vi "GUI_HTT_CTRLv4.vi"() -> ()   [LabVIEW 2020]
uses:
  Shared/GUI_Template/GUI_master/tcp_new_data_event.ctl
  Shared/GUI_Template/GUI_master/tcp new data cluster.ctl
  GUI_TestStand/Fire button.ctl
  <vilib>/Platform/browser.llb/Open URL in Default Browser (string).vi
panel:
  in  "LogEpilog":bool caption="LogTable"
  in  "New Google\nExpLog for new day?":bool=TRUE
  in  "LogTable":bool
  in  "PicoL2":bool caption="PicoL GUI"
  in  "1Wire B GUI":bool caption="PicoL GUI"
  out "fire::12":string="fire" caption="fire"
  in  "Wavelength.Channel0::14":enum16{"248", "355", "532", "800", "2940"}(ring)=enum."532"
  in  "Wavelength.Channel1::14":enum16{"248", "355", "532", "800", "2940"}(ring)=enum."800"
  in  "Wavelength.Channel0::13":enum16{"532", "800"}(ring)=enum."800"
  in  "EnergyRange.Channel0::14":T1(ring)=enum."400mJ"
  in  "EnergyRange.Channel1::14":T1(ring)=enum."400mJ"
  in  "EnergyRange.Channel0::13":T2(ring)=enum."200mJ"
  in  "energy.channel 1::14":dbl caption="Energy Gaia" min=0.0 max=200.0 format="%#_13g"
  out "Energy (J)":dbl
  in  "Multiplicator":dbl=15.3
  in  "GUIdevice 14":string="HTT-Energy-S-G"
  in  "Multiplicator":dbl=66.6
  in  "Multiplicator Scatter":dbl=100.0
  out "Energy Scatter (J)":dbl
  out "Energy (J)":dbl
  in  "energy.channel 0::13":dbl caption="Energy Drive" min=0.0 max=10.0 format="%#_13g"
  in  "energy.channel 0::14":dbl caption="Energy Scatter" min=0.0 max=20.0 format="%#_13g"
  in  "GUIdevice 13":string="HTT-Energy-D"
  in  "IR Pt Exp And Comp":bool caption="PicoL GUI"
  in  "Position.Axis 2::10":dbl caption="y/vert." min=-6000.0 max=6000.0
  in  "Position.Axis 3::10":dbl caption="Scatter Mode z" min=-20.0 max=20.0
  in  "Position.Axis 1::10":dbl caption="x/hor." min=-150.0 max=150.0
  in  "Position.Axis 2::11":dbl caption="Translation" min=-50.0 max=50.0
  in  "Position.Axis 3::11":dbl caption="Rotation G1" min=-360.0 max=360.0
  in  "Position.Axis 1::11":dbl caption="Rotation G2" min=-360.0 max=360.0
  in  "Ethernet Powerstrip":bool caption="Google Drive"
  in  "Position.Axis 3::4":dbl caption="z" min=-10.0 max=26.0
  in  "Position.Axis 2::6":dbl caption="Delay Stage" min=-6000.0 max=6000.0
  in  "FilterWheelB1":bool caption="PicoB GUI"
  in  "Search Log":bool caption="PicoL GUI"
  in  "Experiment \n(if, shadow, topjet)":bool caption="PicoL GUI"
  in  "RemoteDesktop":bool caption="PicoL GUI"
  in  "Experiment \n(e-profile, xrays)":bool caption="PicoL GUI"
  in  "IR TC Pointing (17s)":bool caption="PicoL GUI"
  in  "Scatter Depletion":bool caption="PicoL GUI"
  in  "Scatter IR Amps":bool caption="PicoL GUI"
  in  "Drive TC Pt":bool caption="PicoL GUI"
  in  "Gaia Profiles":bool caption="PicoL GUI"
  in  "Gaia Pointing":bool caption="PicoL GUI"
  in  "IR Exp and Comp":bool caption="PicoL GUI"
  in  "HTT Interactive":bool caption="PicoL GUI"
  in  "GUIdevice 12":string="HTT_DG645"
  in  "Delay.Ch C::12":dbl caption="Delay" min=-0.1 max=2.0 format="%#_6e"
  in  "Delay.Ch D::12":dbl caption="Width" min=-0.1 max=2.0 format="%#_6e"
  in  "Amplitude.Ch CD::12":dbl caption="DG645" min=0.5 max=5.0
  in  "Field::1":dbl caption="B-Field" min=0.0 max=10000.0
  in  "Delay.Ch 1::8":dbl caption="Delay" min=0.0 max=10.0 format="%#_6e"
  in  "Width.Ch 1::8":dbl caption="Width" min=0.0 max=1.0 format="%#_6e"
  in  "Amplitude.Ch 1::8":dbl caption="Cam Trig Amp" min=0.0 max=12.0
  in  "1Wire L GUI":bool caption="PicoL GUI"
  in  "Opt. Spectrometer":bool caption="PicoL GUI"
  in  "SingleCamGUI":bool caption="PicoL GUI"
  in  "Exp Editor":bool caption="PicoL GUI"
  in  "DB Editor":bool caption="PicoL GUI"
  in  "AddColumns":bool caption="PicoL GUI"
  in  "GEECSplot":bool caption="PicoL GUI"
  in  "LVStarter":bool caption="PicoL GUI"
  in  "MasterControl":bool caption="PicoL GUI"
  in  "MagSpecGUI":bool caption="PicoL GUI"
  in  "Google Drive":bool
  in  "Depletion Cams":bool caption="PicoL GUI"
  in  "D-L-Cams":bool caption="PicoL GUI"
  in  "Position.Axis 2::5":dbl caption="Mode Out z" min=-150.0 max=150.0
  in  "Position.Axis 1::4":dbl caption="Blade" min=-20.0 max=20.0
  in  "Amplitude.Ch 5::8":dbl caption="Trigger Amplitude (V)" min=0.0 max=12.0
  in  "Position.Axis 3::5":dbl caption="Drive Mode In z" min=-200.0 max=200.0
  in  "Position.Axis 1::5":dbl caption="Mode Out Wedge" min=-150.0 max=150.0
  out "Position.Axis3::2":dbl caption="Rotation G1" min=-180.0 max=180.0 format="%#_13g"
  out "Position.Axis2::2":dbl caption="Rotation G2" min=-180.0 max=180.0 format="%#_13g"
  in  "Position.Axis1::2":dbl caption="Translation" min=-60000.0 max=60000.0 format="%#_13g"
  in  "PicoL":bool caption="PicoL GUI"
  in  "PicoB":bool caption="PicoB GUI"
  in  "AnalogOutput.Channel 0::9":dbl caption="Pressure Ctrl (V)" min=0.0 max=10.0
  in  "Width.Ch 5::8":dbl caption="Opening time (s)" min=0.0 max=0.025 format="%#_6e"
  in  "Jet enable":bool caption="Jet Enable"
  in  "Jet trigger":bool caption="Jet Trigger"
  in  "Position.Axis 3::3":dbl caption="Jet Z" min=-25.0 max=25.0
  in  "Position.Axis 2::3":dbl caption="Jet Y" min=-25.0 max=25.0
  in  "Position.Axis 1::3":dbl caption="Jet X" min=-25.0 max=25.0
  in  "Position.Axis 3::6":dbl caption="Probe delay" min=-100.0 max=100.0
  in  "GUIdevice 11":string="HTT-ESP05"
  in  "GUIdevice 8":string="HTT-BNC"
  in  "GUIdevice 6":string="HTT-ESP04"
  in  "GUIdevice 5":string="HTT-ESP03"
  in  "Fire Button":T3=TRUE
  out "error IO 2":errorcluster
  out "fire::10":string
  out "tcp data event":T4
  in  "UDP error message":string
  in  "GUIdevice 7":string="HTT-Pulsar"
  in  "GUIdevice 2":string="Aerotech-HTT"
  in  "GUIdevice 10":string="HTT-ESP06"
  in  "GUIdevice 4":string="HTT-ESP02"
  in  "GUIdevice 1":string="HTT-MagTeslameter-DTM141"
  in  "GUIdevice 3":string="HTT-ESP01"
  in  "GUIdevice 9":string="HTT-HighPressureDAQ"
  in  "Delay.Ch 5::8":dbl caption="Jet timing (s)" min=0.0 max=10.0 format="%#_6e"
  in  "stop":bool
  # "Energy"
  # "CAP"
  # "HTT CONTROL CENTER"
  # "v0.5   04/01/2020"
  # "Drive"
  # "Gas Jet"
  # "GUI Collection"
  # "Compressor"
  # "Drive Cameras"
  # "Mode Imager"
  # "Probe Delay Line"
  # "Scatter Cameras"
  # "Scatter"
  # "Compressor"
  # "Electronics"
  # "BNC"
  # "Mode Imager"
  # "Experiment GUIs"
  # "Scatter Delay vs. Drive"
  # "Turning Mirror"
  # "MC Links"
  # "Docu"
  # "Log Maker"
  # "Energy"
  # "Drive"
  # "Scatter"
  # "Gaia"
  # "Adjustment GUIs"
  # "Range"
  # "Wavelength"
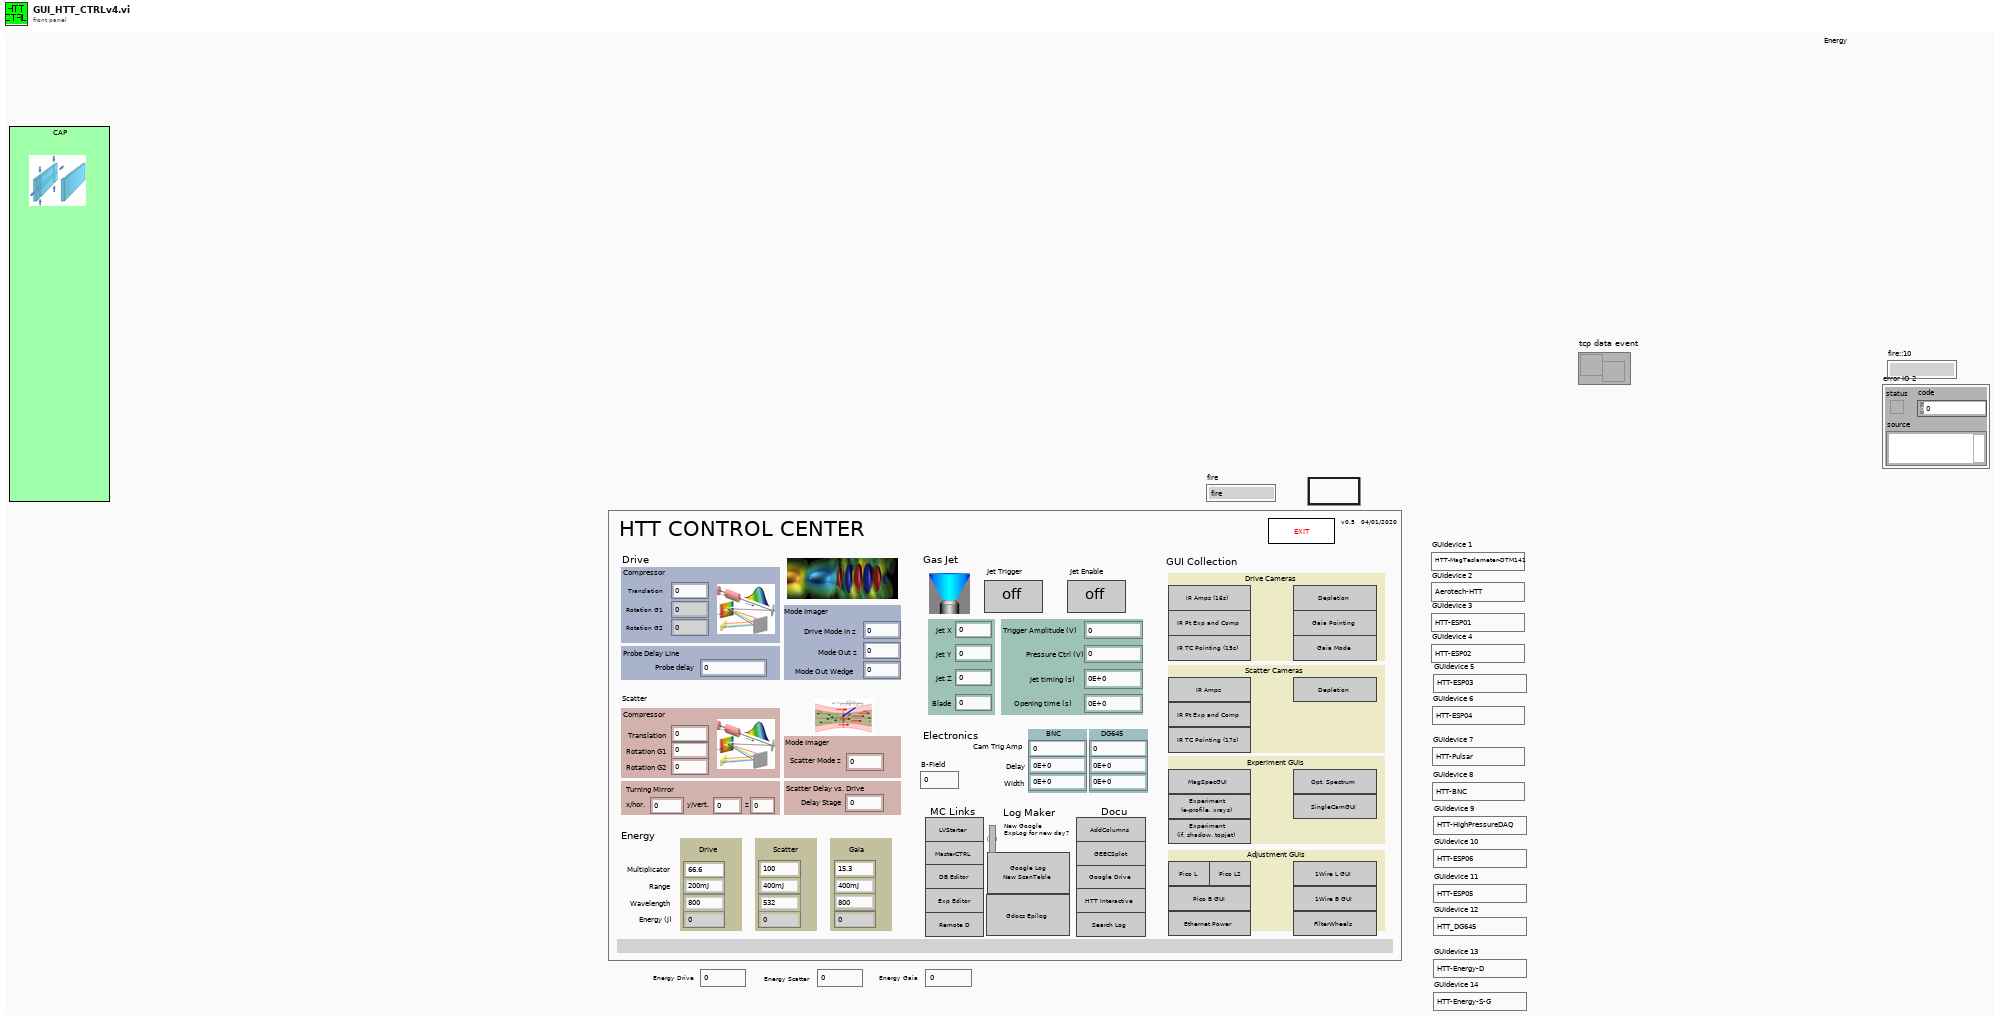
[diagram p1: front panel]
types:
  T1 = enum16{"4.00mJ", "40.0mJ", "400mJ", "4.00J", "20.00J"}
  T2 = enum16{"2.00mJ", "20.0mJ", "200mJ", "2.00J", "10J"}
  T3 = typedef "Fire button.ctl" = bool
  T4 = typedef "tcp_new_data_event.ctl" = refnum<user-event>
  T5 = typedef "tcp new data cluster.ctl" = cluster{"EventEnum":enum16{"new data", "connection status update"}, "Device name":string}
  T6 = enum32{"invalid app kind", "Development System", "Run Time System", "Student Edition", "Embedded LabVIEW", "Evaluation", "Custom"}
  T7 = enum32{"Invalid", "Standard", "Closed", "Hidden", "Minimized", "Maximized"}
  T8 = cluster{"Core":cluster{"Current VI Reference":refnum<vi>, "Close Panel on Exit?":bool}, "Heater timing offset":dbl, "Discharge timing offset":dbl, "Jet trigger":bool, "Tik1":u32, "Tik2":u32, "Fire Continues Allowed":bool, "Jet enable":bool}
  T9 = typedef "imagedata.ctl" = cluster{"image type":i32, "image depth":i32, "image":u8[], "mask":u8[], "colors":u32[], "Rectangle":cluster{"left":i16, "top":i16, "right":i16, "bottom":i16}}
  T10 = cluster{"Current VI Reference":refnum<vi>, "Close Panel on Exit?":bool}
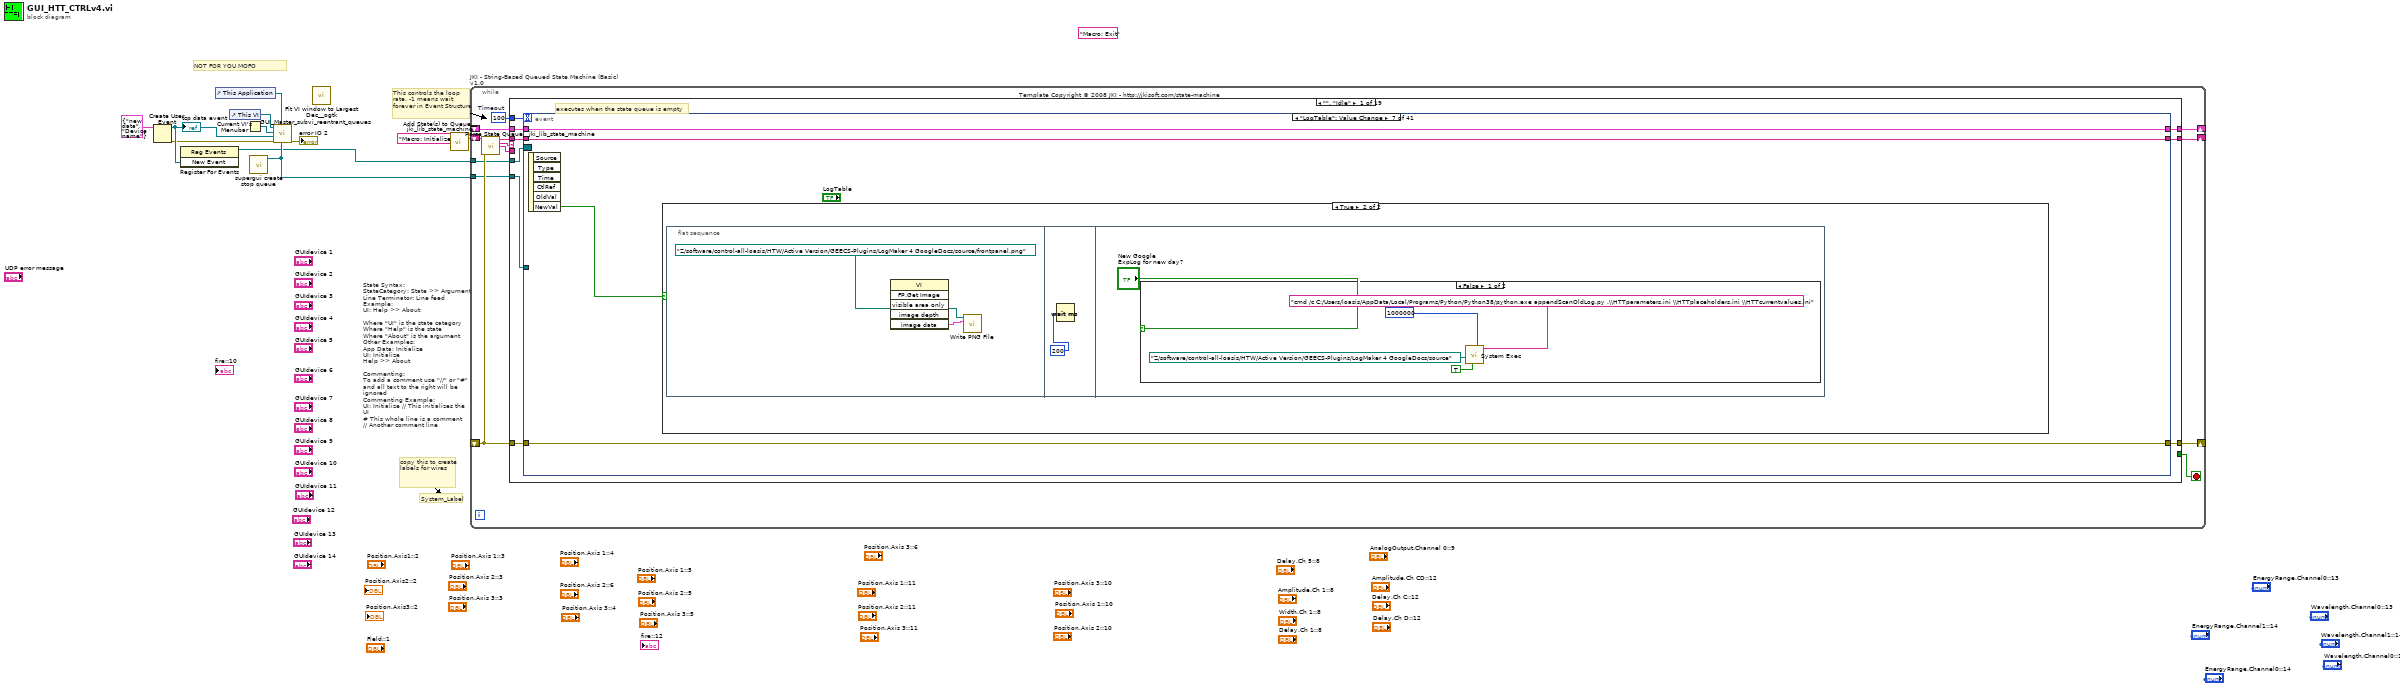
[diagram p0: block diagram]
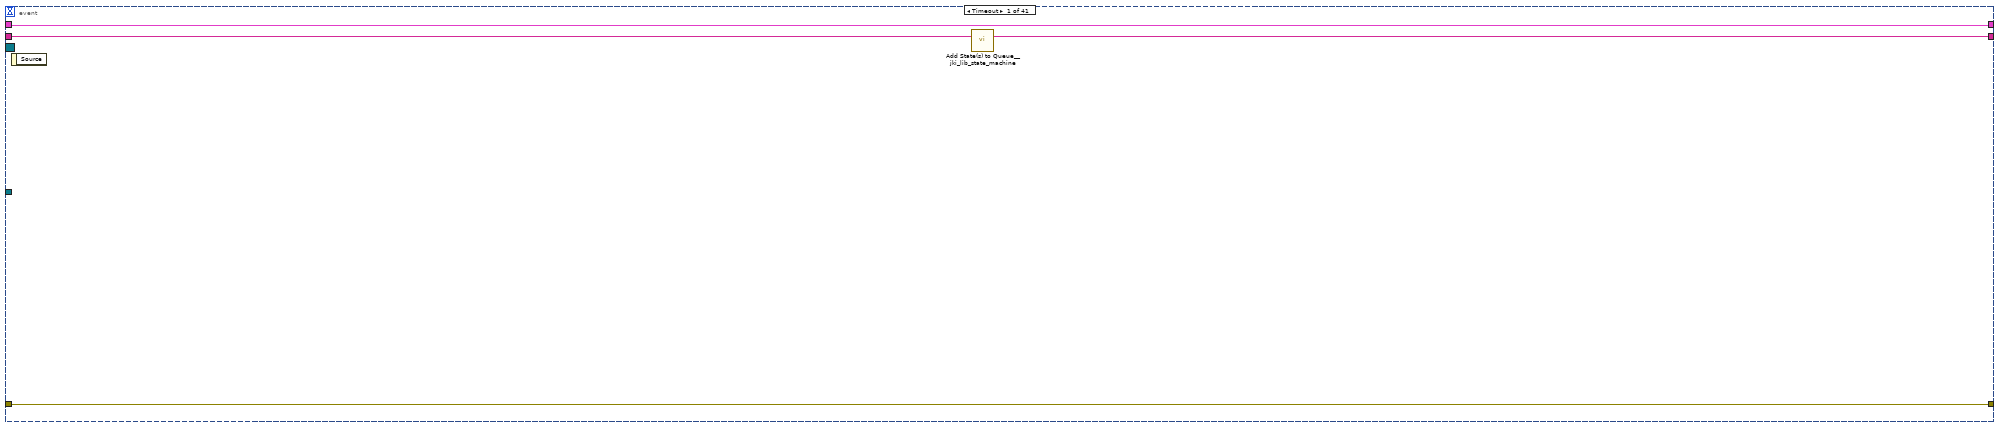
[diagram p2: hidden frame]
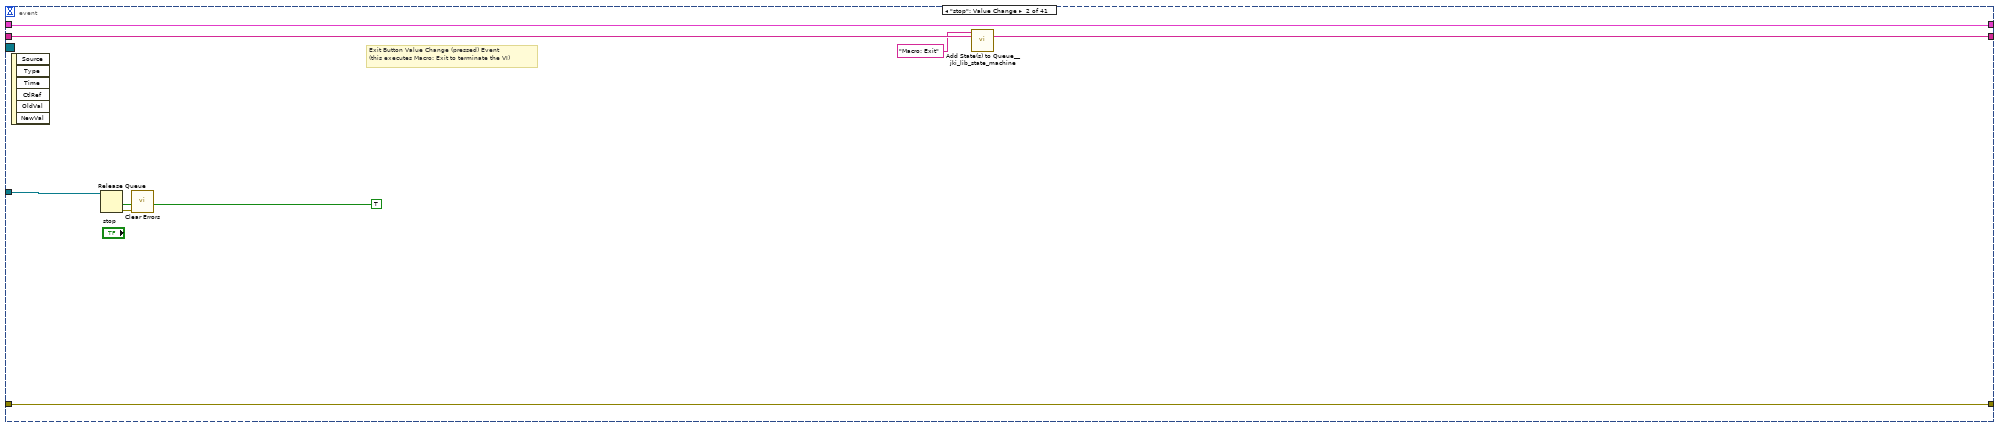
[diagram p3: hidden frame]
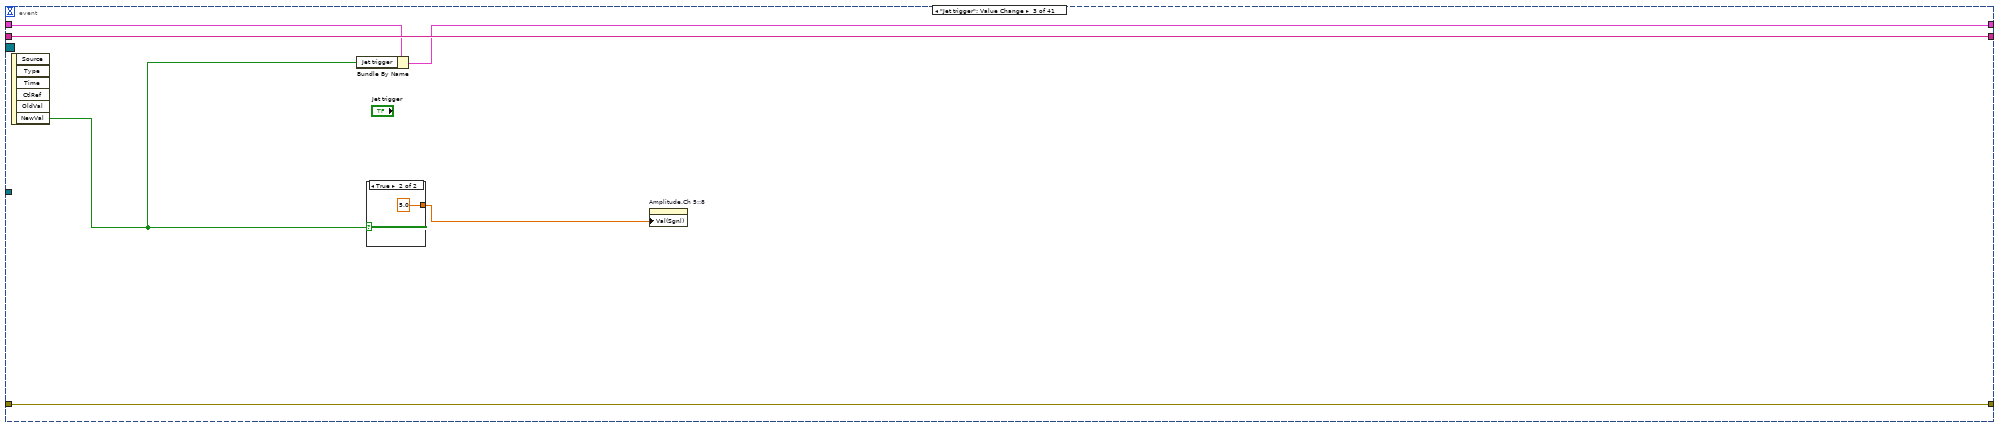
[diagram p4: hidden frame]
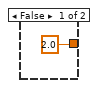
[diagram p5: hidden frame]
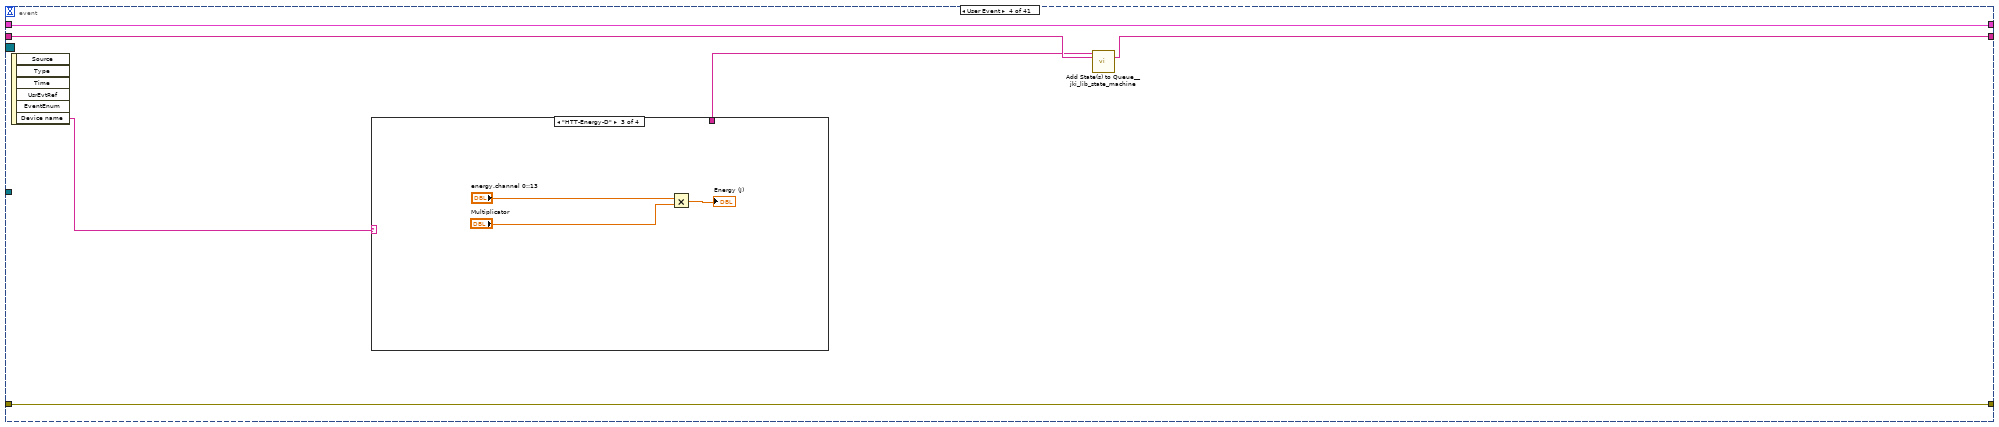
[diagram p6: hidden frame]
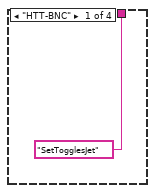
[diagram p7: hidden frame]
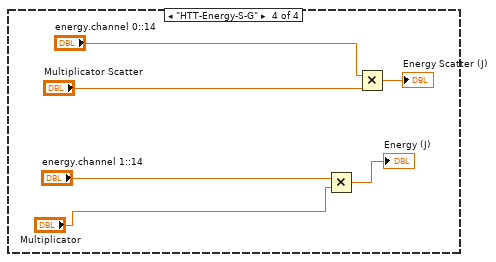
[diagram p9: hidden frame]
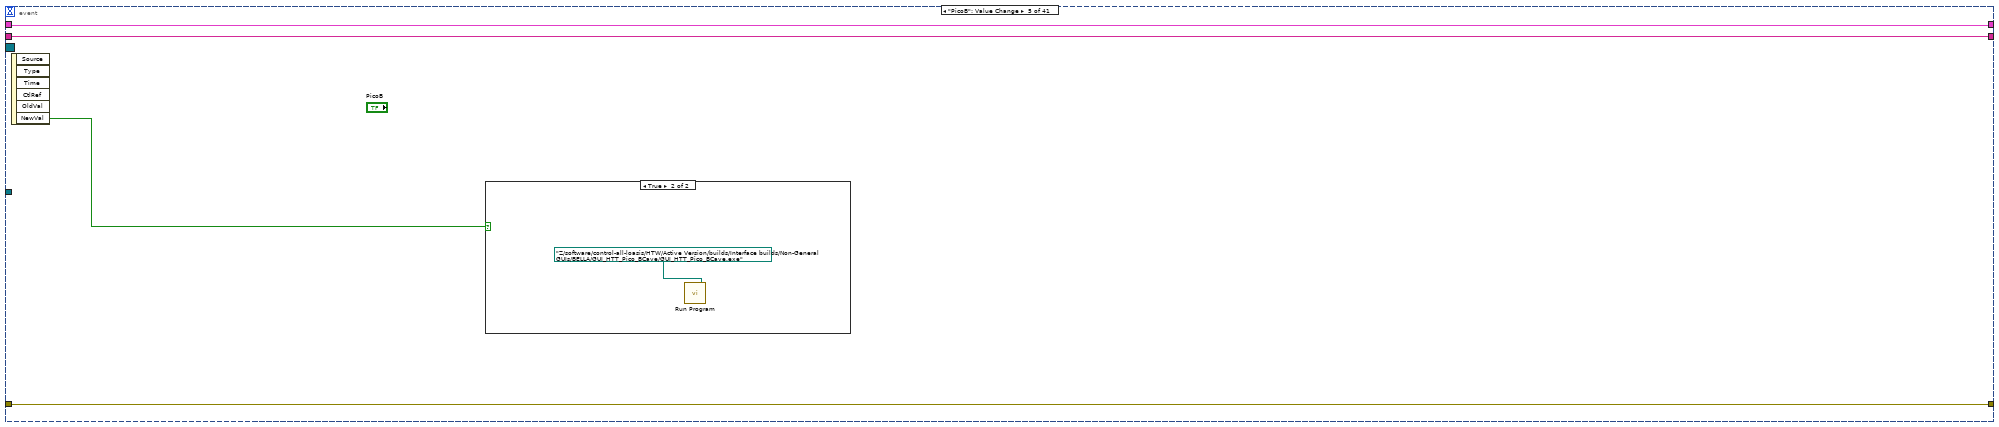
[diagram p10: hidden frame]
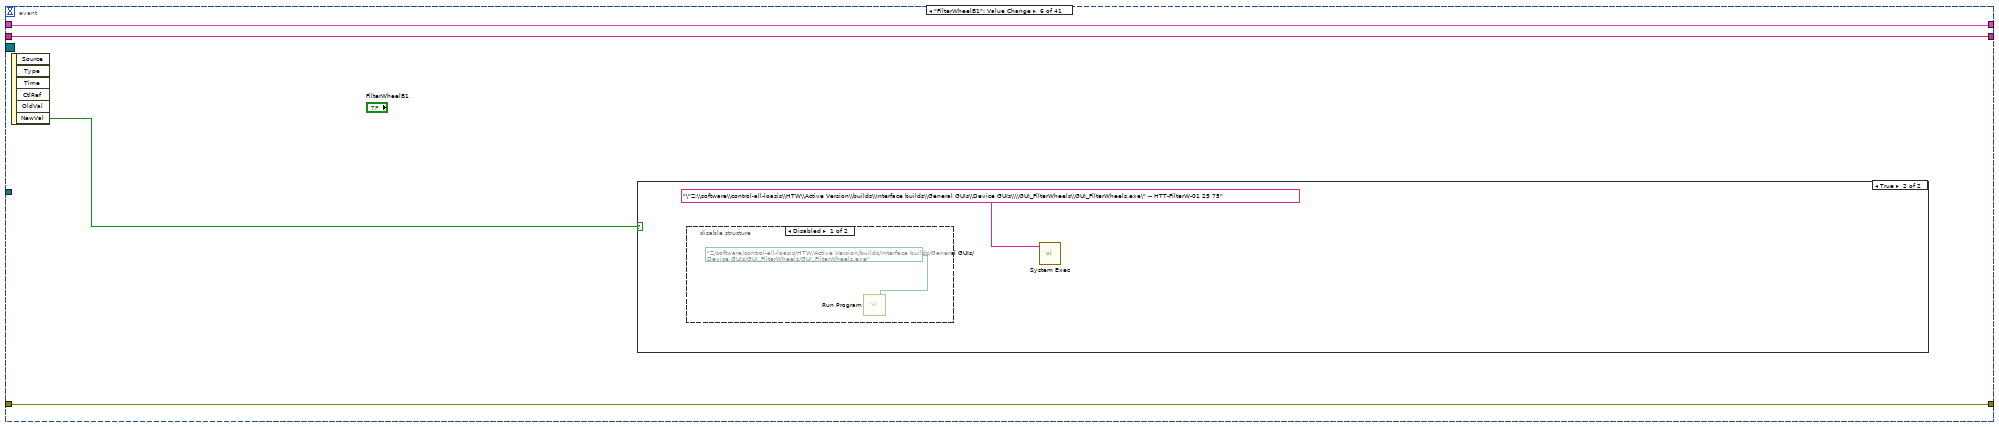
[diagram p12: hidden frame]
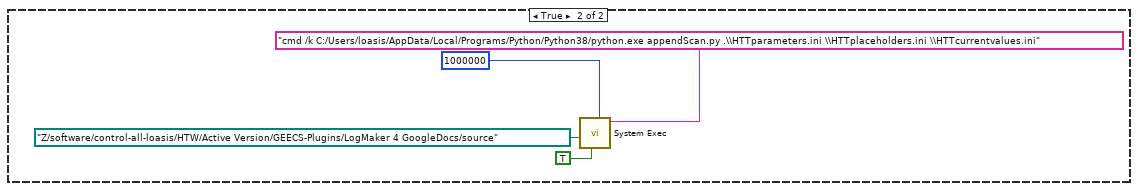
[diagram p16: hidden frame]
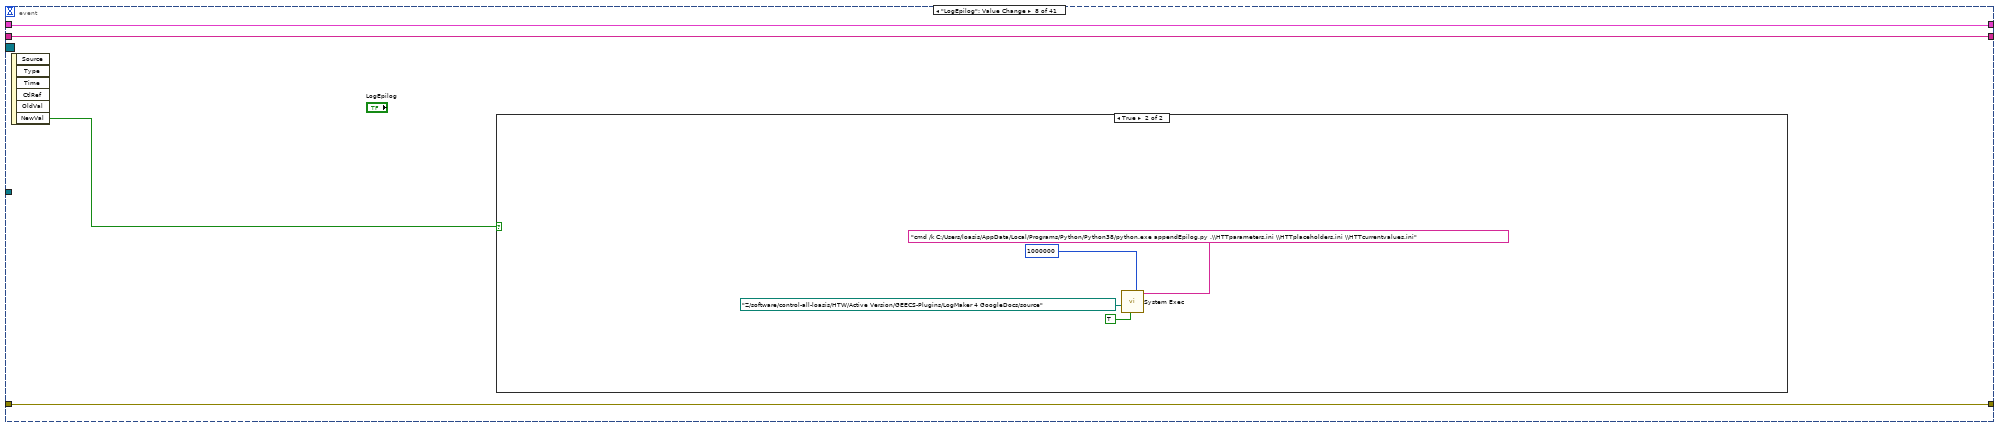
[diagram p17: hidden frame]
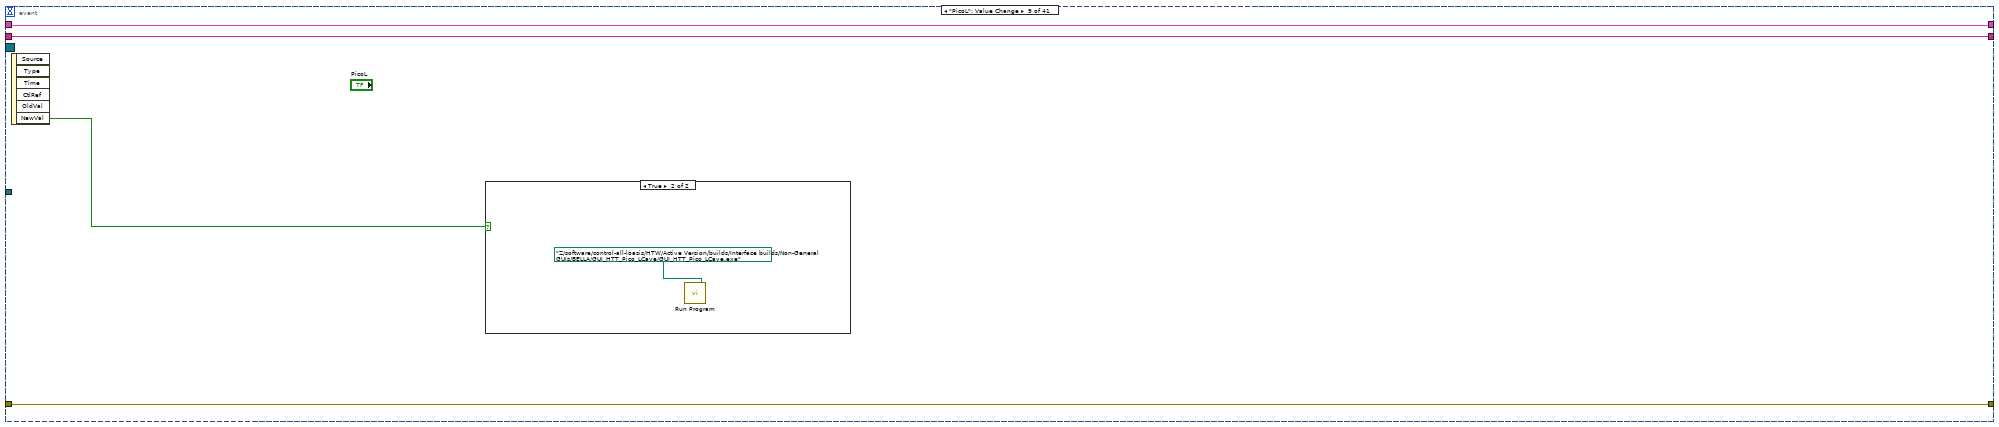
[diagram p19: hidden frame]
diagram:
  (unwired) "Macro: Exit"
  # "State Syntax:\nStateCategory: State >> Argument\nLine Terminator: Line feed\nExample:\nUI: Help >> About\n\nWhere \"UI\" is the state category\nWhere \"Help\" is the state\nWhere \"About\" is the argument\nOther Examples:\nApp Data: Initialize\nUI: Initialize\nHelp >> About\n\nCommenting:\nTo add a comment use \"//\" or \"#\" and all text to the right will be ignored\nCommenting Example:\nUI: Initialize // This initializes the UI\n# This whole line is a comment\n// Another comment line"
  # "copy this to create labels for wires"
  # "This controls the loop rate. -1 means wait forever in Event Structure"
  # "System_Label"
  # "NOT FOR YOU MOFO"
  n1 = Create User Event(user event datatype=T5 {"EventEnum"=enum."new data", "Device name"="Device name"} ("New Event")) -> (user event=w10:refnum<user-event>, error out=w9:errorcluster)  [unwired: 1 in]
  "tcp data event" <- w10
  n2 = register-events(w10) -> (reference out=w1:refnum<event-registration>)  [unwired: 2 in, 1 out]
  n3 = control-ref of="This Application"() -> (w11:refnum<vi>)
  n4 = control-ref of="This VI"() -> (w5:refnum<vi>)
  n5 = Current VI's Menubar() -> (w7:refnum<k9>)
  n6 = call "supergui create stop queue.vi"() -> ("STOP Queue out"=w2:refnum<queue>)  [unwired: 11 in]
  n7 = call "GUI_Master_subvi_reentrant_queues.vi"("STOP Queue in"=w2, "This Application"=w11, "error in (no error)"=w9, "tcp data event"=w10, "Caller menu reference"=w7, "Caller VI ref"=w5) -> ("error out"=→"error IO 2":errorcluster)  [unwired: 5 in]
  n8 = call <userlib>:"Fit VI window to Largest Dec__ogtk.vi"() -> ()  [unwired: 6 in, 2 out]
  n9 = call <vilib>:"Add State(s) to Queue__jki_lib_state_machine.vi"("State(s) in (\"\")"="Macro: Initialize") -> ("States Out"=w3:string)  [unwired: 14 in]
  n10 = while "JKI - String-Based Queued State Machine (Basic) v1.0" {
    shift-right: [w18] -> _
    shift-left: _ -> [w17]
    shift-right: [w20] -> _
    shift-left: _ -> [w15]
    shift-right: [w19] -> _
    shift-left: w3 -> [w21]
    tunnel: w1 -> [w14]
    tunnel: w2 -> [w13]
    stop <- w12 stop-if-true
    w16 = 100  # Timeout
    # "Template Copyright © 2008 JKI - http://jkisoft.com/state-machine"
    n11 = call <vilib>:"Parse State Queue__jki_lib_state_machine.vi"("State Queue"=w21, "Error In (no error)"=w15) -> ("Remaining States"=w23:string, "Current State"=w24:string, "Arguments"=w22:string)  [unwired: 11 in]
    n12 = case shown="\"\", \"Idle\"" w24 {
      selector: w24 -> [_ _ _ w294 _ _ _ _ _ _ _ _ _ _ _ _ _ _ _]
      tunnel: w23 -> [w33 w288 w293 w298 w316 w322 w327 w331 w343 w349 w353 w357 w363 w374 w400 w405 w415 w419 w425]
      tunnel: w22 -> [_ _ _ _ _ _ _ _ _ _ _ _ w358 w368 _ _ _ _ _]
      tunnel: w17 -> [w31 w289 w290 w296 w307 w319 w325 w328 _ w344 w350 w355 w361 w370 w397 w402 w412 w416 w423]
      tunnel: [w30 w287 w291 w300 w313 errorcluster {"status"=FALSE, "code"=0, "source"=""} ("error out") w324 w329 w340 w345 w351 w354 w359 w371 w398 w403 w413 w417 w420] -> w20
      tunnel: w15 -> [w29 w287 w291 w299 w313 w318 w324 w329 w340 w346 w351 w354 w360 w372 w398 w403 w413 w417 w421]
      tunnel: [w32 w288 w292 w297 w315 w321 w326 w330 w342 w348 w352 w356 w362 w373 w399 w404 w414 w418 w424] -> w19
      tunnel: [_ _ _ _ _ _ TRUE _ _ _ _ _ _ _ _ _ _ _ _] -> w12
      tunnel: [w25 w289 w290 w296 w314 w319 w325 w328 w341 w344 w350 w355 w361 w370 w397 w402 w412 w416 w423] -> w18
      tunnel: w16 -> [w28 _ _ _ _ _ _ _ _ _ _ _ _ _ _ _ _ _ _]
      tunnel: w14 -> [w27 _ _ _ _ _ _ _ _ _ _ _ _ _ _ _ _ _ _]
      tunnel: w13 -> [w26 _ _ _ _ _ _ _ _ _ _ _ _ _ _ _ _ _ _]
      frame "", "Idle" {
        # "executes when the state queue is empty"
        n13 = event shown="[6] \"LogTable\": Value Change" {
          selector: w27 -> [_ _ _ _ _ _ _ _ _ _ _ _ _ _ _ _ _ _ _ _ _ _ _ _ _ _ _ _ _ _ _ _ _ _ _ _ _ _ _ _ _]
          dyn-events: _ -> [_ _ _ _ _ _ _ _ _ _ _ _ _ _ _ _ _ _ _ _ _ _ _ _ _ _ _ _ _ _ _ _ _ _ _ _ _ _ _ _ _]
          timeout: w28 -> [_ _ _ _ _ _ _ _ _ _ _ _ _ _ _ _ _ _ _ _ _ _ _ _ _ _ _ _ _ _ _ _ _ _ _ _ _ _ _ _ _]
          tunnel: w33 -> [w37 w45 w51 w57 w73 w78 w84 w100 w108 w113 w118 w123 w128 w133 w138 w143 w148 w153 w158 w163 w168 w173 w178 w183 w188 w193 w198 w203 w208 w213 w218 w223 w228 w233 w238 w243 w248 w253 w260 w265 w274]
          tunnel: [w36 w44 w51 w56 w73 w78 w84 w100 w108 w113 w118 w123 w128 w133 w138 w143 w148 w153 w158 w163 w168 w173 w178 w183 w188 w193 w198 w203 w208 w213 w218 w223 w228 w233 w238 w243 w248 w253 w260 w266 w273] -> w32
          tunnel: w31 -> [w34 w42 w50 w58 w70 w75 w81 w97 w105 w110 w115 w120 w125 w130 w135 w140 w145 w150 w155 w160 w165 w170 w175 w180 w185 w190 w195 w200 w205 w210 w215 w220 w225 w230 w235 w240 w245 w250 w259 w268 w271]
          tunnel: [w35 w43 w47 w55 w71 w76 w82 w98 w106 w111 w116 w121 w126 w131 w136 w141 w146 w151 w156 w161 w166 w171 w176 w181 w186 w191 w196 w201 w206 w211 w216 w221 w226 w231 w236 w241 w246 w251 w255 w267 w272] -> w30
          tunnel: w29 -> [w35 w43 w47 w55 w71 w76 w82 w98 w106 w111 w116 w121 w126 w131 w136 w141 w146 w151 w156 w161 w166 w171 w176 w181 w186 w191 w196 w201 w206 w211 w216 w221 w226 w231 w236 w241 w246 w251 w255 w267 w272]
          tunnel: [w34 w42 w49 w58 w70 w75 w81 w97 w105 w110 w115 w120 w125 w130 w135 w140 w145 w150 w155 w160 w165 w170 w175 w180 w185 w190 w195 w200 w205 w210 w215 w220 w225 w230 w235 w240 w245 w250 w258 w268 w271] -> w25
          tunnel: w26 -> [_ w39 _ _ _ _ _ _ _ _ _ _ _ _ _ _ _ _ _ _ _ _ _ _ _ _ _ _ _ _ _ _ _ _ _ _ _ _ _ _ _]
          event Timeout {
            n14 = event-data() -> ()  [unwired: 1 in, 1 out]
            n15 = call <vilib>:"Add State(s) to Queue__jki_lib_state_machine.vi"("State(s) in (\"\")"=w37) -> ("States Out"=w36:string)  [unwired: 14 in]
          }
          event "stop": Value Change {
            # "Exit Button Value Change (pressed) Event\n(this executes Macro: Exit to terminate the VI)"
            n16 = event-data() -> ()  [unwired: 1 in, 6 out]
            n17 = Release Queue(queue=w39, force destroy? (F)=TRUE) -> (error out=w40:errorcluster)  [unwired: 1 in, 2 out]
            n18 = call <vilib>:"Clear Errors.vi"("error in (no error)"=w40) -> ()  [unwired: 5 in, 2 out]
            n19 = call <vilib>:"Add State(s) to Queue__jki_lib_state_machine.vi"("State(s) in Front (\"\")"="Macro: Exit", "State(s) in (\"\")"=w45) -> ("States Out"=w44:string)  [unwired: 13 in]
          }
          event "Jet trigger": Value Change {
            n20 = event-data() -> ("NewVal"=w48:bool)  [unwired: 1 in, 5 out]
            n21 = Bundle By Name(cluster=w50, "Jet trigger"=w48) -> (w49:T8)
            n22 = case shown="True" w48 {
              tunnel: [2.0 ("Amplitude.Ch CD::10") 5.0 ("Amplitude.Ch CD::10")] -> w46
              frame False {
              }
              frame True {
              }
            }
            n23 = property on="Amplitude.Ch 5::8" class="DigNum (strict)"("Val(Sgnl)"=w46) -> ()  [unwired: 2 in, 2 out]
          }
          event User Event {
            n24 = event-data() -> ("Device name"=w59:string)  [unwired: 1 in, 5 out]
            n25 = case shown="\"HTT-Energy-D\"" w59 {
              tunnel: ["SetTogglesJet" _ _ _] -> w54
              frame "HTT-BNC" {
              }
              frame "False", Default {
              }
              frame "HTT-Energy-D" {
                n26 = Multiply(x="energy.channel 0::13", y="Multiplicator") -> (x*y=→"Energy (J)":dbl)
              }
              frame "HTT-Energy-S-G" {
                n27 = Multiply(x="energy.channel 1::14", y="Multiplicator") -> (x*y=→"Energy (J)":dbl)
                n28 = Multiply(x="energy.channel 0::14", y="Multiplicator Scatter") -> (x*y=→"Energy Scatter (J)":dbl)
              }
            }
            n29 = call <vilib>:"Add State(s) to Queue__jki_lib_state_machine.vi"("State(s) in Front (\"\")"=w54, "State(s) in (\"\")"=w57) -> ("States Out"=w56:string)  [unwired: 13 in]
          }
          event "PicoB": Value Change {
            n30 = event-data() -> ("NewVal"=w72:bool)  [unwired: 1 in, 5 out]
            n31 = case shown="True" w72 {
              frame False {
              }
              frame True {
                n32 = call "Run Program.vi"("Program Path"=path "Z:/software/control-all-loasis/HTW/Active Version/builds/Interface builds/Non-General GUIs/BELLA/GUI_HTT_Pico_BCave/GUI_HTT_Pico_BCave.exe") -> ()  [unwired: 1 in]
              }
            }
          }
          event "FilterWheelB1": Value Change {
            n33 = event-data() -> ("NewVal"=w77:bool)  [unwired: 1 in, 5 out]
            n34 = case shown="True" w77 {
              frame False {
              }
              frame True {
                n35 = disable-structure shown="Disabled" {
                  frame Disabled {
                    n36 = call "Run Program.vi"("Program Path"=path "Z:/software/control-all-loasis/HTW/Active Version/builds/Interface builds/General GUIs/Device GUIs/GUI_FilterWheels/GUI_FilterWheels.exe") -> ()  [unwired: 1 in]
                  }
                  frame Enabled {
                  }
                }
                n37 = call <vilib>:"System Exec.vi"("command line"="\"Z:\\software\\control-all-loasis\\HTW\\Active Version\\builds\\Interface builds\\General GUIs\\Device GUIs\\\\GUI_FilterWheels\\GUI_FilterWheels.exe\" -- HTT-FilterW-01 25 75") -> ()  [unwired: 7 in, 4 out]
              }
            }
          }
          event "LogTable": Value Change {
            n38 = event-data() -> ("NewVal"=w83:bool)  [unwired: 1 in, 5 out]
            n39 = case shown="True" w83 {
              frame False {
              }
              frame True {
                n40 = flat-sequence {
                  frame #0 {
                    n41 = invoke class="VI" method="FP.Get Image"() -> ("image data"=w86:T9)  [unwired: 6 in, 5 out]
                    n42 = call <vilib>:"Write PNG File.vi"("image data"=w86, "path to PNG file"=path "Z:/software/control-all-loasis/HTW/Active Version/GEECS-Plugins/LogMaker 4 GoogleDocs/source/frontpanel.png" ("report file path")) -> ()  [unwired: 8 in, 2 out]
                  }
                  frame #1 {
                    n43 = Wait (ms)(milliseconds to wait=u32 200 ("millisecond timer value")) -> ()  [unwired: 1 out]
                  }
                  frame #2 {
                    n44 = case shown="False" "New Google\nExpLog for new day?" {
                      frame False {
                        n45 = call <vilib>:"System Exec.vi"("expected output size  (4096)"=u32 1000000, "run minimized? (F)"=TRUE, "working directory"=path "Z:/software/control-all-loasis/HTW/Active Version/GEECS-Plugins/LogMaker 4 GoogleDocs/source", "command line"="cmd /c C:/Users/loasis/AppData/Local/Programs/Python/Python38/python.exe appendScanOldLog.py .\\HTTparameters.ini \\HTTplaceholders.ini \\HTTcurrentvalues.ini") -> ()  [unwired: 4 in, 4 out]
                      }
                      frame True {
                        n46 = call <vilib>:"System Exec.vi"("expected output size  (4096)"=u32 1000000, "run minimized? (F)"=TRUE, "working directory"=path "Z:/software/control-all-loasis/HTW/Active Version/GEECS-Plugins/LogMaker 4 GoogleDocs/source", "command line"="cmd /k C:/Users/loasis/AppData/Local/Programs/Python/Python38/python.exe appendScan.py .\\HTTparameters.ini \\HTTplaceholders.ini \\HTTcurrentvalues.ini") -> ()  [unwired: 4 in, 4 out]
                      }
                    }
                  }
                }
              }
            }
          }
          event "LogEpilog": Value Change {
            n47 = event-data() -> ("NewVal"=w99:bool)  [unwired: 1 in, 5 out]
            n48 = case shown="True" w99 {
              frame False {
              }
              frame True {
                n49 = call <vilib>:"System Exec.vi"("expected output size  (4096)"=u32 1000000, "run minimized? (F)"=TRUE, "working directory"=path "Z:/software/control-all-loasis/HTW/Active Version/GEECS-Plugins/LogMaker 4 GoogleDocs/source", "command line"="cmd /k C:/Users/loasis/AppData/Local/Programs/Python/Python38/python.exe appendEpilog.py .\\HTTparameters.ini \\HTTplaceholders.ini \\HTTcurrentvalues.ini") -> ()  [unwired: 4 in, 4 out]
              }
            }
          }
          event "PicoL": Value Change {
            n50 = event-data() -> ("NewVal"=w107:bool)  [unwired: 1 in, 5 out]
            n51 = case shown="True" w107 {
              frame False {
              }
              frame True {
                n52 = call "Run Program.vi"("Program Path"=path "Z:/software/control-all-loasis/HTW/Active Version/builds/Interface builds/Non-General GUIs/BELLA/GUI_HTT_Pico_LCave/GUI_HTT_Pico_LCave.exe") -> ()  [unwired: 1 in]
              }
            }
          }
          event "PicoL2": Value Change {
            n53 = event-data() -> ("NewVal"=w112:bool)  [unwired: 1 in, 5 out]
            n54 = case shown="True" w112 {
              frame False {
              }
              frame True {
                n55 = call "Run Program.vi"("Program Path"=path "Z:/software/control-all-loasis/HTW/Active Version/builds/Interface builds/Non-General GUIs/BELLA/GUI_HTT_Pico_LCave2/GUI_HTT_Pico_LCave2.exe") -> ()  [unwired: 1 in]
              }
            }
          }
          event "D-L-Cams": Value Change {
            n56 = event-data() -> ("NewVal"=w117:bool)  [unwired: 1 in, 5 out]
            n57 = case shown="True" w117 {
              frame False {
              }
              frame True {
                n58 = call "Run Program.vi"("Program Path"=path "Z:/software/control-all-loasis/HTW/Active Version/builds/Interface builds/Non-General GUIs/BELLA/GUI_HTT_MultiCam/GUI_HTT_MultiCamsDriveAmp.exe") -> ()  [unwired: 1 in]
              }
            }
          }
          event "Depletion Cams": Value Change {
            n59 = event-data() -> ("NewVal"=w122:bool)  [unwired: 1 in, 5 out]
            n60 = case shown="True" w122 {
              frame False {
              }
              frame True {
                n61 = call "Run Program.vi"("Program Path"=path "Z:/software/control-all-loasis/HTW/Active Version/builds/Interface builds/Non-General GUIs/BELLA/GUI_HTT_MultiCam/GUI_HTT_MultiCamsDriveDepletion.exe") -> ()  [unwired: 1 in]
              }
            }
          }
          event "Gaia Profiles": Value Change {
            n62 = event-data() -> ("NewVal"=w127:bool)  [unwired: 1 in, 5 out]
            n63 = case shown="True" w127 {
              frame False {
              }
              frame True {
                n64 = call "Run Program.vi"("Program Path"=path "Z:/software/control-all-loasis/HTW/Active Version/builds/Interface builds/Non-General GUIs/BELLA/GUI_HTT_MultiCam/GUI_HTT_MultiCamsDriveGaiaProfile.exe") -> ()  [unwired: 1 in]
              }
            }
          }
          event "Drive TC Pt": Value Change {
            n65 = event-data() -> ("NewVal"=w132:bool)  [unwired: 1 in, 5 out]
            n66 = case shown="True" w132 {
              frame False {
              }
              frame True {
                n67 = call "Run Program.vi"("Program Path"=path "Z:/software/control-all-loasis/HTW/Active Version/builds/Interface builds/Non-General GUIs/BELLA/GUI_HTT_MultiCam/GUI_HTT_MultiCamsDriveTCPointing.exe") -> ()  [unwired: 1 in]
              }
            }
          }
          event "Scatter IR Amps": Value Change {
            n68 = event-data() -> ("NewVal"=w137:bool)  [unwired: 1 in, 5 out]
            n69 = case shown="True" w137 {
              frame False {
              }
              frame True {
                n70 = call "Run Program.vi"("Program Path"=path "Z:/software/control-all-loasis/HTW/Active Version/builds/Interface builds/Non-General GUIs/BELLA/GUI_HTT_MultiCam/GUI_HTT_MultiCamsScatterAmp.exe") -> ()  [unwired: 1 in]
              }
            }
          }
          event "Scatter Depletion": Value Change {
            n71 = event-data() -> ("NewVal"=w142:bool)  [unwired: 1 in, 5 out]
            n72 = case shown="True" w142 {
              frame False {
              }
              frame True {
                n73 = call "Run Program.vi"("Program Path"=path "Z:/software/control-all-loasis/HTW/Active Version/builds/Interface builds/Non-General GUIs/BELLA/GUI_HTT_MultiCam/GUI_HTT_MultiCamsScatterDepletion.exe") -> ()  [unwired: 1 in]
              }
            }
          }
          event "IR Exp and Comp": Value Change {
            n74 = event-data() -> ("NewVal"=w147:bool)  [unwired: 1 in, 5 out]
            n75 = case shown="True" w147 {
              frame False {
              }
              frame True {
                n76 = call "Run Program.vi"("Program Path"=path "Z:/software/control-all-loasis/HTW/Active Version/builds/Interface builds/Non-General GUIs/BELLA/GUI_HTT_MultiCam/GUI_HTT_MultiCamsDriveExpAndComp.exe") -> ()  [unwired: 1 in]
              }
            }
          }
          event "Gaia Pointing": Value Change {
            n77 = event-data() -> ("NewVal"=w152:bool)  [unwired: 1 in, 5 out]
            n78 = case shown="True" w152 {
              frame False {
              }
              frame True {
                n79 = call "Run Program.vi"("Program Path"=path "Z:/software/control-all-loasis/HTW/Active Version/builds/Interface builds/Non-General GUIs/BELLA/GUI_HTT_MultiCam/GUI_HTT_MultiCamsDriveGaiaPointing.exe") -> ()  [unwired: 1 in]
              }
            }
          }
          event "1Wire L GUI": Value Change {
            n80 = event-data() -> ("NewVal"=w157:bool)  [unwired: 1 in, 5 out]
            n81 = case shown="True" w157 {
              frame False {
              }
              frame True {
                n82 = call "Run Program.vi"("Program Path"=path "Z:/software/control-all-loasis/HTW/Active Version/builds/Interface builds/Non-General GUIs/BELLA/GUI_HTT_1Wire/GUI_HTT_1Wire.exe") -> ()  [unwired: 1 in]
              }
            }
          }
          event "1Wire B GUI": Value Change {
            n83 = event-data() -> ("NewVal"=w162:bool)  [unwired: 1 in, 5 out]
            n84 = case shown="True" w162 {
              frame False {
              }
              frame True {
                n85 = call "Run Program.vi"("Program Path"=path "Z:/software/control-all-loasis/HTW/Active Version/builds/Interface builds/Non-General GUIs/BELLA/GUI_HTT_1Wire_BCave/GUI_HTT_1Wire_BCave.exe") -> ()  [unwired: 1 in]
              }
            }
          }
          event "MagSpecGUI": Value Change {
            n86 = event-data() -> ("NewVal"=w167:bool)  [unwired: 1 in, 5 out]
            n87 = case shown="True" w167 {
              frame False {
              }
              frame True {
                n88 = call "Run Program.vi"("Program Path"=path "Z:/software/control-all-loasis/HTW/Active Version/builds/Interface builds/Non-General GUIs/BELLA/GUI_HTT_MultiCam/GUI_HTT_MultiCamsDriveMagSpec.exe") -> ()  [unwired: 1 in]
              }
            }
          }
          event "IR TC Pointing (17s)": Value Change {
            n89 = event-data() -> ("NewVal"=w172:bool)  [unwired: 1 in, 5 out]
            n90 = case shown="True" w172 {
              frame False {
              }
              frame True {
                n91 = call "Run Program.vi"("Program Path"=path "Z:/software/control-all-loasis/HTW/Active Version/builds/Interface builds/Non-General GUIs/BELLA/GUI_HTT_MultiCam/GUI_HTT_MultiCamsScatterTCPointing.exe") -> ()  [unwired: 1 in]
              }
            }
          }
          event "IR Pt Exp And Comp": Value Change {
            n92 = event-data() -> ("NewVal"=w177:bool)  [unwired: 1 in, 5 out]
            n93 = case shown="True" w177 {
              frame False {
              }
              frame True {
                n94 = call "Run Program.vi"("Program Path"=path "Z:/software/control-all-loasis/HTW/Active Version/builds/Interface builds/Non-General GUIs/BELLA/GUI_HTT_MultiCam/GUI_HTT_MultiCamsScatterExpAndComp.exe") -> ()  [unwired: 1 in]
              }
            }
          }
          event "Experiment \n(e-profile, xrays)": Value Change {
            n95 = event-data() -> ("NewVal"=w182:bool)  [unwired: 1 in, 5 out]
            n96 = case shown="True" w182 {
              frame False {
              }
              frame True {
                n97 = call "Run Program.vi"("Program Path"=path "Z:/software/control-all-loasis/HTW/Active Version/builds/Interface builds/Non-General GUIs/BELLA/GUI_HTT_MultiCam/GUI_HTT_MultiCamsDriveExperiment1.exe") -> ()  [unwired: 1 in]
              }
            }
          }
          event "Experiment \n(if, shadow, topjet)": Value Change {
            n98 = event-data() -> ("NewVal"=w187:bool)  [unwired: 1 in, 5 out]
            n99 = case shown="True" w187 {
              frame False {
              }
              frame True {
                n100 = call "Run Program.vi"("Program Path"=path "Z:/software/control-all-loasis/HTW/Active Version/builds/Interface builds/Non-General GUIs/BELLA/GUI_HTT_MultiCam/GUI_HTT_MultiCamsDriveExperiment2.exe") -> ()  [unwired: 1 in]
              }
            }
          }
          event "MasterControl": Value Change {
            n101 = event-data() -> ("NewVal"=w192:bool)  [unwired: 1 in, 5 out]
            n102 = case shown="True" w192 {
              frame False {
              }
              frame True {
                n103 = call "Run Program.vi"("Program Path"=path "Z:/software/control-all-loasis/HTW/Active Version/builds/Interface builds/General GUIs/MC/Master Control/Master Control.exe") -> ()  [unwired: 1 in]
              }
            }
          }
          event "LVStarter": Value Change {
            n104 = event-data() -> ("NewVal"=w197:bool)  [unwired: 1 in, 5 out]
            n105 = case shown="True" w197 {
              frame False {
              }
              frame True {
                n106 = call "Run Program.vi"("Program Path"=path "Z:/software/control-all-loasis/HTW/Active Version/builds/Interface builds/General GUIs/MC/LVstarter/LVstarter.exe") -> ()  [unwired: 1 in]
              }
            }
          }
          event "GEECSplot": Value Change {
            n107 = event-data() -> ("NewVal"=w202:bool)  [unwired: 1 in, 5 out]
            n108 = case shown="True" w202 {
              frame False {
              }
              frame True {
                n109 = call "Run Program.vi"("Program Path"=path "P:/10_Software/ajg builds/GEECSplotter 20200129/GEECSplotter.exe") -> ()  [unwired: 1 in]
              }
            }
          }
          event "AddColumns": Value Change {
            n110 = event-data() -> ("NewVal"=w207:bool)  [unwired: 1 in, 5 out]
            n111 = case shown="True" w207 {
              frame False {
              }
              frame True {
                n112 = call "Run Program.vi"("Program Path"=path "P:/10_Software/ajg builds/Add columns to Masterlog 20200213/Add columns to Masterlog.exe") -> ()  [unwired: 1 in]
              }
            }
          }
          event "DB Editor": Value Change {
            n113 = event-data() -> ("NewVal"=w212:bool)  [unwired: 1 in, 5 out]
            n114 = case shown="True" w212 {
              frame False {
              }
              frame True {
                n115 = call "Run Program.vi"("Program Path"=path "Z:/software/control-all-loasis/HTW/Active Version/builds/Interface builds/General GUIs/Database editor/Database editor.exe") -> ()  [unwired: 1 in]
              }
            }
          }
          event "Exp Editor": Value Change {
            n116 = event-data() -> ("NewVal"=w217:bool)  [unwired: 1 in, 5 out]
            n117 = case shown="True" w217 {
              frame False {
              }
              frame True {
                n118 = call "Run Program.vi"("Program Path"=path "Z:/software/control-all-loasis/HTW/Active Version/builds/Interface builds/General GUIs/Database editor/Expt_Devices_GUI_Datagridview.exe") -> ()  [unwired: 1 in]
              }
            }
          }
          event "SingleCamGUI": Value Change {
            n119 = event-data() -> ("NewVal"=w222:bool)  [unwired: 1 in, 5 out]
            n120 = case shown="True" w222 {
              frame False {
              }
              frame True {
                n121 = call "Run Program.vi"("Program Path"=path "Z:/software/control-all-loasis/HTW/Active Version/builds/Interface builds/General GUIs/Device GUIs/GUI_Cameras/GUI_Cameras.exe") -> ()  [unwired: 1 in]
              }
            }
          }
          event "Opt. Spectrometer": Value Change {
            n122 = event-data() -> ("NewVal"=w227:bool)  [unwired: 1 in, 5 out]
            n123 = case shown="True" w227 {
              frame False {
              }
              frame True {
                n124 = call "Run Program.vi"("Program Path"=path "Z:/software/control-all-loasis/HTW/Active Version/builds/Interface builds/Non-General GUIs/BELLA/GUI_HTT_HamamatsuSpec/GUI_HTT_HamamatsuSpec.exe") -> ()  [unwired: 1 in]
              }
            }
          }
          event "RemoteDesktop": Value Change {
            n125 = event-data() -> ("NewVal"=w232:bool)  [unwired: 1 in, 5 out]
            n126 = case shown="True" w232 {
              frame False {
              }
              frame True {
                n127 = call "Run Program.vi"("Program Path"=path "C:/Windows/System32/mstsc.exe") -> ()  [unwired: 1 in]
              }
            }
          }
          event "Google Drive": Value Change {
            n128 = event-data() -> ("NewVal"=w237:bool)  [unwired: 1 in, 5 out]
            n129 = case shown="True" w237 {
              frame False {
              }
              frame True {
                # "HTT daily ops"
                n130 = call-poly <vilib>:"Open URL in Default Browser.vi"("URL"="https://drive.google.com/drive/folders/0B6BJlLNDz1MaOC10bXdFbHFBQ00?usp=sharing") -> ()  [unwired: 5 in, 2 out]
              }
            }
          }
          event "Ethernet Powerstrip": Value Change {
            n131 = event-data() -> ("NewVal"=w242:bool)  [unwired: 1 in, 5 out]
            n132 = case shown="True" w242 {
              frame False {
              }
              frame True {
                # "Ethernet Powerstrip"
                n133 = call-poly <vilib>:"Open URL in Default Browser.vi"("URL"="http://192.168.7.229/outlet.html") -> ()  [unwired: 5 in, 2 out]
              }
            }
          }
          event "HTT Interactive": Value Change {
            n134 = event-data() -> ("NewVal"=w247:bool)  [unwired: 1 in, 5 out]
            n135 = case shown="True" w247 {
              frame False {
              }
              frame True {
                n136 = call-poly <vilib>:"Open URL in Default Browser.vi"("URL"="https://docs.google.com/presentation/d/1vde03GLRziloe-kxBmiBfXX4-hwSL2uU9dDMmq9JgxY/edit?usp=sharing") -> ()  [unwired: 5 in, 2 out]
              }
            }
          }
          event "Search Log": Value Change {
            n137 = event-data() -> ("NewVal"=w252:bool)  [unwired: 1 in, 5 out]
            n138 = case shown="True" w252 {
              frame False {
              }
              frame True {
                n139 = call-poly <vilib>:"Open URL in Default Browser.vi"("URL"="https://docs.google.com/spreadsheets/d/1wR7To7WJHrQNP-2Id8ScCGPPim0LYwsaw_KNOLmAjJY/edit?usp=sharing") -> ()  [unwired: 5 in, 2 out]
              }
            }
          }
          event "Jet enable": Value Change {
            # "For instructions on how to use the JKI State Machine, examples and video tutorials, visit:\nhttp://jkisoft.com/state-machine/\n\nJKI State Machine™\nhttp://jkisoft.com/state-machine/\nCopyright (C) 2005-2008, JKI <info@jkisoft.com>\nALL RIGHTS RESERVED"
            n140 = event-data() -> ("NewVal"=w257:bool)  [unwired: 1 in, 5 out]
            n141 = case shown="True" w257 {
              tunnel: [0.0 ("opening Time") 0.002 ("opening Time")] -> w256
              frame False {
              }
              frame True {
              }
            }
            n142 = Bundle By Name(cluster=w259, "Jet enable"=w257) -> (w258:T8)
            n143 = property on="Width.Ch 5::8" class="DigNum (strict)"("Val(Sgnl)"=w256) -> ()  [unwired: 2 in, 2 out]
          }
          event Value Change {
            n144 = event-data() -> ()  [unwired: 1 in, 6 out]
            n145 = property on="fire::12" class="Str"("Val(Sgnl)"="fire>>force" ("Value (Signaling)")) -> ()  [unwired: 2 in, 2 out]
            n146 = call <vilib>:"Add State(s) to Queue__jki_lib_state_machine.vi"("State(s) in Front (\"\")"="Action: Fire" ("State(s) in Front (\"\")"), "State(s) in (\"\")"=w265) -> ("States Out"=w266:string)  [unwired: 13 in]
          }
          event Panel Close? {
            # "Discard the event because we'll close the front panel ourselves in Macro: Exit"
            # "Close Panel button (pressed) Event\n(this executes Macro: Exit to terminate the VI)"
            n147 = event-data() -> ()  [unwired: 1 in, 1 out]
            n148 = call <vilib>:"Add State(s) to Queue__jki_lib_state_machine.vi"("State(s) in Front (\"\")"="Macro: Exit", "State(s) in (\"\")"=w274) -> ("States Out"=w273:string)  [unwired: 13 in]
            n149 = event-data("Discard?"=TRUE) -> ()  [unwired: 1 in, 1 out]
          }
        }
      }
      frame "SetTogglesJet" {
        n150 = Greater?(x="Amplitude.Ch 5::8", y=2.5) -> (0:w284:bool)
        n151 = Select(t=TRUE, s=w284, f=FALSE) -> (s? t:f=w281:bool)
        n152 = Greater?(x="Width.Ch 5::8", y=0.0001) -> (0:w276:bool)
        n153 = Select(t=TRUE, s=w276, f=FALSE) -> (s? t:f=w275:bool)
        n154 = local write "Jet enable"(w275) -> ()
        n155 = local write "Jet trigger"(w281) -> ()
      }
      frame "---------- Core ----------" {
        # "Do not put any code in this frame.\n(it is a separator no-op)"
        n156 = call <vilib>:"Add State(s) to Queue__jki_lib_state_machine.vi"("State(s) in (\"\")"=w293) -> ("States Out"=w292:string)  [unwired: 14 in]
      }
      frame Default {
        w303 = 42 items=["No error", "Argument error", "Memory is full", "Out of zone", "End of file", "File already open", "Generic file I/O error", "File not found", "File permission error", "Disk is full", "Duplicate path", "Too many files open", "System feature not enabled", "Resource file not found", "Cannot add resource", "Resource not found", "Image not found", "Image memory error", "Pen does not exist", "Config type invalid", "Config token not found", "Config parse error", "Config memory error", "Bad external code format", "Bad external code offset", "External code not present", "Null window", "Destroy window error", "Null menu", "Print aborted", "Bad print record", "Print driver error", "Windows error during printing", "Memory error during printing", "Print dialog error", "Generic print error", "Invalid device refnum", "Device not found", "Device parameter error", "Device unit error", "Cannot open device", "Device call aborted", "Generic error", "Cancelled by user", "Object ID too low", "Object ID too high", "Object not in heap", "Unknown heap", "Unknown object (invalid DefProc)", "Unknown object (DefProc not in table)", "Message out of range", "Invalid (null) method", "Unknown message", "Manager call not supported", "Bad address", "Network operation in progress", "Network operation timed out", "Connection is busy", "Network attribute not supported", "Network error", "Address in use", "System out of memory", "Connection aborted", "Connection refused", "Not connected", "Already connected", "Connection closed", "Initialization error (interapplication manager)", "Bad occurrence", "Wait on unbound occurrence handler", "Occurrence queue overflow", "Datalog type conflict", "Unused", "Unrecognized type (interapplication manager)", "Memory corrupt", "Failed to make temporary DLL", "Old CIN version", "Drag socket not found", "Failed to load drop-object", "Failed to register OLE object", "Failed to release OLE object", "Format specifier type mismatch", "Unknown format specifier", "Too few format specifiers", "Too many format specifiers", "Scan failed", "Newer CIN version", "Error converting to variant", "Runtime menu error", "Password tampered", "Variant attribute not found", "Incompatible variant data type", "Event data is not available", "Event Store is not present", "Occurrence is not found", "Event Queue is not created", "Event info is not available", "Refnum passed is NULL", "Error retrieving Class GUID", "Error retrieving CoClass GUID", "Error retrieving TypeLib GUID.", "Bad built application magic bytes.", "Specific driver is different from the specific driver associated with the Logical Name.", "There is no session opened to the class driver.", "Max Error", "MAX - Error with config objects", "MAX - Error loading configuration", "MAX - Group not supported"]
        # "Current State"
        # "Do not delete, rename, or modify this frame.\n(this is used to capture unhandled states and typos)"
        # "Handle mistyped state name (developer tool)"
        n157 = Format Into String(format string="Software Exception: Unhandled State \"%s\"." ("message"), error in=w299, w294) -> (resulting string=w302:string, error out=w301:errorcluster)  [unwired: 1 in]
        n158 = call <vilib>:"Error Cluster From Error Code.vi"("show call chain? (False)"=TRUE, "error in (no error)"=w301, "error message (\"\")"=w302, "error code (0)"=w303) -> ("error out"=w300:errorcluster)  [unwired: 5 in]
        n159 = call <vilib>:"Add State(s) to Queue__jki_lib_state_machine.vi"("State(s) in (\"\")"=w298) -> ("States Out"=w297:string)  [unwired: 14 in]
      }
      frame "Initialize Core Data" {
        # "Do not delete, rename, or modify this frame.\n(this is used to determine panel behavior on exit)"
        # "originally closed?"
        # "exe?"
        # "If panel starts closed or is an EXE, then close it when we exit"
        n160 = property class="VI"() -> ("Front Panel.Open"=w312:bool)  [unwired: 2 in, 2 out]
        n161 = property class="App"() -> ("App.Kind"=w311:T6)  [unwired: 2 in, 2 out]
        n162 = control-ref of="Current VI Reference"() -> (w305:refnum<vi>)
        n163 = Not(x=w312) -> (.not. x?=w309:bool)
        n164 = Equal?(x=w311, y=T6."Run Time System" ("Application:Kind")) -> (x = y?=w308:bool)
        n165 = Or(x=w309, y=w308) -> (x .or. y?=w306:bool)
        n166 = Bundle By Name(cluster=w307, "Core.Current VI Reference"=w305, "Core.Close Panel on Exit?"=w306) -> (w314:T8)
        n167 = call <vilib>:"Add State(s) to Queue__jki_lib_state_machine.vi"("State(s) in (\"\")"=w316) -> ("States Out"=w315:string)  [unwired: 14 in]
      }
      frame "Error Handler" {
        # "Unhandled Error -- Display it"
        # "Handle any errors here.\nYou can also output any states to clean-up after errors occur"
        # "Clear error"
        n168 = call <vilib>:"General Error Handler.vi"("error in (no error)"=w318) -> ()  [unwired: 10 in, 5 out]
        n169 = call <vilib>:"Add State(s) to Queue__jki_lib_state_machine.vi"("State(s) in Front (\"\")"="/* Post Error States", "State(s) in (\"\")"=w322) -> ("States Out"=w321:string)  [unwired: 13 in]
      }
      frame "Exit" {
        # "Do not put any code in this frame.\n(No errors that occur here will be handled.)"
        n170 = call <vilib>:"Add State(s) to Queue__jki_lib_state_machine.vi"("State(s) in (\"\")"=w327) -> ("States Out"=w326:string)  [unwired: 14 in]
      }
      frame "---------- Data ----------" {
        # "Do not put any code in this frame.\n(It is a separator no-op. You can make a copy of this frame to create a new Data frame)"
        n171 = call <vilib>:"Add State(s) to Queue__jki_lib_state_machine.vi"("State(s) in (\"\")"=w331) -> ("States Out"=w330:string)  [unwired: 14 in]
      }
      frame "Data: Initialize" {
        w332 = FALSE  # Jet enable
        w333 = FALSE  # Fire Continues Allowed
        w335 = u32 0  # Tik1
        w334 = u32 0  # Tik2
        w336 = FALSE  # Jet trigger
        w337 = 0.0  # Discharge timing offset
        w338 = 0.0  # Heater timing offset
        w339 = T10 {"Current VI Reference"=refnum, "Close Panel on Exit?"=FALSE}  # Core
        # "do not delete - used by framework"
        # "Expand Bundle to add new data elements to shift register data."
        # "Add new data here."
        # "Data names and types of shift register data are defined by this bundle."
        # "Initialize the shift-register data, here.\n(data names are defined by what you wire into the bundle function)"
        n172 = Bundle("Core"=w339, "Heater timing offset"=w338, "Discharge timing offset"=w337, "Jet trigger"=w336, "Tik1"=w335, "Tik2"=w334, "Fire Continues Allowed"=w333, "Jet enable"=w332) -> (w341:T8)  [unwired: 1 in]
        n173 = call <vilib>:"Add State(s) to Queue__jki_lib_state_machine.vi"("State(s) in (\"\")"=w343) -> ("States Out"=w342:string)  [unwired: 14 in]
      }
      frame "Data: Cleanup" {
        # "Cleanup any data and references, here.\n(this is called automatically, by the Macro: Exit)"
        n174 = Unbundle By Name(w344) -> ("Core.Current VI Reference"=w347:refnum<vi>)
        n175 = Close Reference(reference=w347, error in (no error)=w346) -> (error out=w345:errorcluster)
        n176 = call <vilib>:"Add State(s) to Queue__jki_lib_state_machine.vi"("State(s) in (\"\")"=w349) -> ("States Out"=w348:string)  [unwired: 14 in]
      }
      frame "---------- UI ----------" {
        # "Do not put any code in this frame.\n(It is a separator no-op. You can make a copy of this frame to create a new UI frame)"
        n177 = call <vilib>:"Add State(s) to Queue__jki_lib_state_machine.vi"("State(s) in (\"\")"=w353) -> ("States Out"=w352:string)  [unwired: 14 in]
      }
      frame "UI: Initialize" {
        # "Initialize the User Interface, here.\n(this is called automatically, by the Macro: Init)"
        n178 = call <vilib>:"Add State(s) to Queue__jki_lib_state_machine.vi"("State(s) in (\"\")"=w357) -> ("States Out"=w356:string)  [unwired: 14 in]
      }
      frame "UI: Cursor Set" {
        # "Argument"
        # "Set and Unset Cursor Busy.\n(Usage: \"UI: Cursor Set >> Busy|Idle\")"
        n179 = case shown="\"Idle\", Default" w358 {
          tunnel: w360 -> [w365 w367]
          tunnel: [w364 w366] -> w359
          frame "Idle", Default {
            n180 = call <vilib>:"Unset Busy.vi"("error in (no error)"=w365) -> ("error out"=w364:errorcluster)  [unwired: 10 in]
          }
          frame "Busy" {
            n181 = call <vilib>:"Set Busy.vi"("error in (no error)"=w367) -> ("error out"=w366:errorcluster)  [unwired: 9 in, 1 out]
          }
        }
        n182 = call <vilib>:"Add State(s) to Queue__jki_lib_state_machine.vi"("State(s) in (\"\")"=w363) -> ("States Out"=w362:string)  [unwired: 14 in]
      }
      frame "UI: Front Panel State" {
        # "Argument"
        # "Set Front Panel Open or Closed\n(Usage: \"UI: Front Panel State >> Open|Close\")"
        n183 = Unbundle By Name(w370) -> ("Core.Current VI Reference"=w369:refnum<vi>)
        n184 = case shown="\"Close\"" w368 {
          tunnel: w372 -> [w378 w391]
          tunnel: [w380 w392] -> w371
          tunnel: w369 -> [w379 w389]
          frame "Open", Default {
            n185 = property class="VI"(reference=w379, error in=w378) -> (reference out=w376:refnum<vi>, error out=w377:errorcluster, "Front Panel.Open"=w375:bool)
            n186 = case shown="False" w375 {
              tunnel: [w383 w386] -> w380
              tunnel: w377 -> [w382 w386]
              tunnel: w376 -> [w381 _]
              frame False {
                n187 = invoke class="VI" method="FP.Open"(reference=w381, error in=w382, "Activate"=TRUE, "State"=T7."Standard") -> (error out=w383:errorcluster)  [unwired: 1 in, 4 out]
              }
              frame True {
              }
            }
          }
          frame "Close" {
            n188 = property class="VI"(reference=w389, error in=w391) -> (reference out=w388:refnum<vi>, error out=w390:errorcluster, "Front Panel.Open"=w387:bool)
            n189 = case shown="True" w387 {
              tunnel: [w393 w396] -> w392
              tunnel: w390 -> [w393 w395]
              tunnel: w388 -> [_ w394]
              frame False {
              }
              frame True {
                n190 = invoke class="VI" method="FP.Close"(reference=w394, error in=w395) -> (error out=w396:errorcluster)  [unwired: 1 in, 2 out]
              }
            }
          }
        }
        n191 = call <vilib>:"Add State(s) to Queue__jki_lib_state_machine.vi"("State(s) in (\"\")"=w374) -> ("States Out"=w373:string)  [unwired: 14 in]
      }
      frame "---------- Macro ----------" {
        # "Do not put any code in this frame.\n(It is a separator no-op. You can make a copy of this frame to create a new Macro frame)"
        n192 = call <vilib>:"Add State(s) to Queue__jki_lib_state_machine.vi"("State(s) in (\"\")"=w400) -> ("States Out"=w399:string)  [unwired: 14 in]
      }
      frame "Macro: Initialize" {
        w401 = "Data: Initialize\nInitialize Core Data\nUI: Initialize\nUI: Front Panel State >> Open"  # Data: Initialize Initialize Core Data UI: Initialize UI: Front Panel State >> Open
        # "Initialization Macro\n(This is called once, when the VI starts)"
        n193 = call <vilib>:"Add State(s) to Queue__jki_lib_state_machine.vi"("State(s) in Front (\"\")"=w401, "State(s) in (\"\")"=w405) -> ("States Out"=w404:string)  [unwired: 13 in]
      }
      frame "Macro: Exit" {
        # "Exit Macro\n(This is called once, when the VI exits)"
        n194 = Unbundle By Name(w412) -> ("Core.Close Panel on Exit?"=w411:bool)
        n195 = Select(t="UI: Front Panel State >> Close", s=w411, f="") -> (s? t:f=w408:string)
        n196 = call <vilib>:"Add State(s) to Queue__jki_lib_state_machine.vi"("State(s) in (\"\")"=w408, "State(s) at Back (\"\")"="Data: Cleanup\nExit") -> ("States Out"=w406:string)  [unwired: 13 in]
        n197 = call <vilib>:"Add State(s) to Queue__jki_lib_state_machine.vi"("State(s) in Front (\"\")"=w406, "State(s) in (\"\")"=w415) -> ("States Out"=w414:string)  [unwired: 13 in]
      }
      frame "---------- New Category ----------" {
        # "Template Separator\n(You can make a copy of, or modify, this frame)"
        n198 = call <vilib>:"Add State(s) to Queue__jki_lib_state_machine.vi"("State(s) in (\"\")"=w419) -> ("States Out"=w418:string)  [unwired: 14 in]
      }
      frame "Action: Fire" {
        # "Your code here.\n(You can make a copy of, or modify, this frame)"
        n199 = property on="fire::10" class="Str"(error in=w421, "Val(Sgnl)"="fire>>force" ("Value (Signaling)")) -> (error out=w420:errorcluster)  [unwired: 1 in, 1 out]
        n200 = call <vilib>:"Add State(s) to Queue__jki_lib_state_machine.vi"("State(s) in (\"\")"=w425) -> ("States Out"=w424:string)  [unwired: 14 in]
      }
    }
  }
